vi "Array mean & Coefficient of Variation.vi"(11 "Data":dbl[](array[numeric])) -> (1 "Coeffecient of variation":dbl, 3 "Mean":dbl format="%0.2f")   [LabVIEW 2020]
uses:
  <vilib>/Analysis/NI_AALBase.lvlib
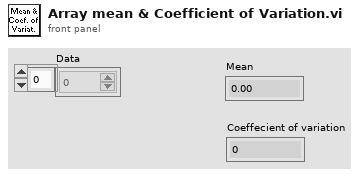
[diagram p1: front panel]
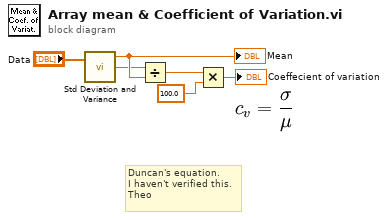
[diagram p0: block diagram]
diagram:
  # "Duncan's equation.\nI haven't verified this.\nTheo"
  n1 = call <vilib>:"Std Deviation and Variance.vi"("X"="Data") -> ("mean"=w5:dbl, "standard deviation"=w3:dbl)  [unwired: 1 in, 1 out]
  "Mean" <- w5
  n2 = Divide(x=w3, y=w5) -> (x/y=w2:dbl)
  n3 = Multiply(x=w2, y=100.0) -> (x*y=→"Coeffecient of variation":dbl)
